vi "Keithley2450GateS.vi"() -> ()   [LabVIEW 2025]
doc: "Author: Scott Hannahs <sth@magnet.fsu.edu>\n\nThis software is licensed for use under the “MIT License\"\nCopyright (c) 2025 Scott Hannahs, sth@sth@magnet.sthnet.net\n\nPermission is hereby granted, free of charge, to any person obtaining a copy of this software and associated documentation files (the \"Software\"), to deal in the Software without restriction, including without limitation the rights to use, copy, modify, merge, publish, distribute, sublicense, and/or sell copies of the Software, and to permit persons to whom the Software is furnished to do so, subject to the following conditions: The above copyright notice and this permission notice shall be included in all copies or substantial portions of the Software.\n\nTHE SOFTWARE IS PROVIDED \"AS IS\", WITHOUT WARRANTY OF ANY KIND, EXPRESS OR IMPLIED, INCLUDING BUT NOT LIMITED TO THE WARRANTIES OF MERCHANTABILITY, FITNESS FOR A PARTICULAR PURPOSE AND NONINFRINGEMENT. IN NO EVENT SHALL THE AUTHORS OR COPYRIGHT HOLDERS BE LIABLE FOR ANY CLAIM, DAMAGES OR OTHER LIABILITY, WHETHER IN AN ACTION OF CONTRACT, TORT OR OTHERWISE, ARISING FROM, OUT OF OR IN CONNECTION WITH THE SOFTWARE OR THE USE OR OTHER DEALINGS IN THE SOFTWARE."
panel:
  out "Sweep\nTime  (sec)":u32 format="%.1f"
  in  "Button:SetupBySoft":bool
  in  "Autozero:":bool
  out "Was paused":bool=TRUE
  in  "VISA resource name":refnum<visa-resource-name>="GPIB0::15::INSTR"
  in  "INFINITE RUN":bool
  in  "MODE:":enum32{"SAW /|/|/|", "TRINGLE /\\/\\/\\"}(radio)=enum."TRINGLE /\\/\\/\\"
  in  "Step |Volt| (abs.)":dbl=0.05 min=1e-06 max=0.1 format="%^.3e"
  in  "Delay (s)":dbl=1.0 min=0.1 max=100.0 format="%.3f"
  in  "Stop Volt":dbl=1.0 min=-10.0 max=10.0 format="%^.3e"
  in  "Start Sweep":bool
  out "Last index":i32
  in  "Compliance Current":dbl=1e-07 format="%.3e"
  in  "Start Volt":dbl min=-10.0 max=10.0 format="%^.3e"
  in  "Setup":bool
  in  "Pause/Resume sweep":bool
  out "StartStorage":dbl min=-10.0 max=10.0 format="%^.3e"
  out "StopStorage":dbl=1.0 min=-10.0 max=10.0 format="%^.3e"
  in  "Button:Continue":bool
  in  "Button:SweepBySoft":bool
  out "Volt by Computer":dbl min=-10.0 max=10.0 format="%^.3e"
  in  "stop sweep":bool
  in  "Output Zero":bool
  # "Select name then start VI"
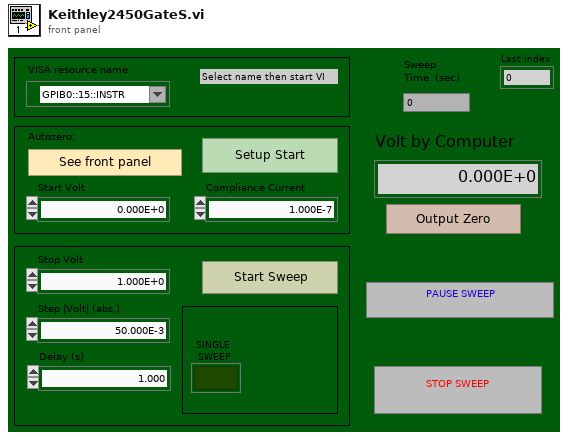
[diagram p1: front panel]
types:
  T1 = enum8{"Enabled", "Disabled", "Disabled and Grayed Out"}
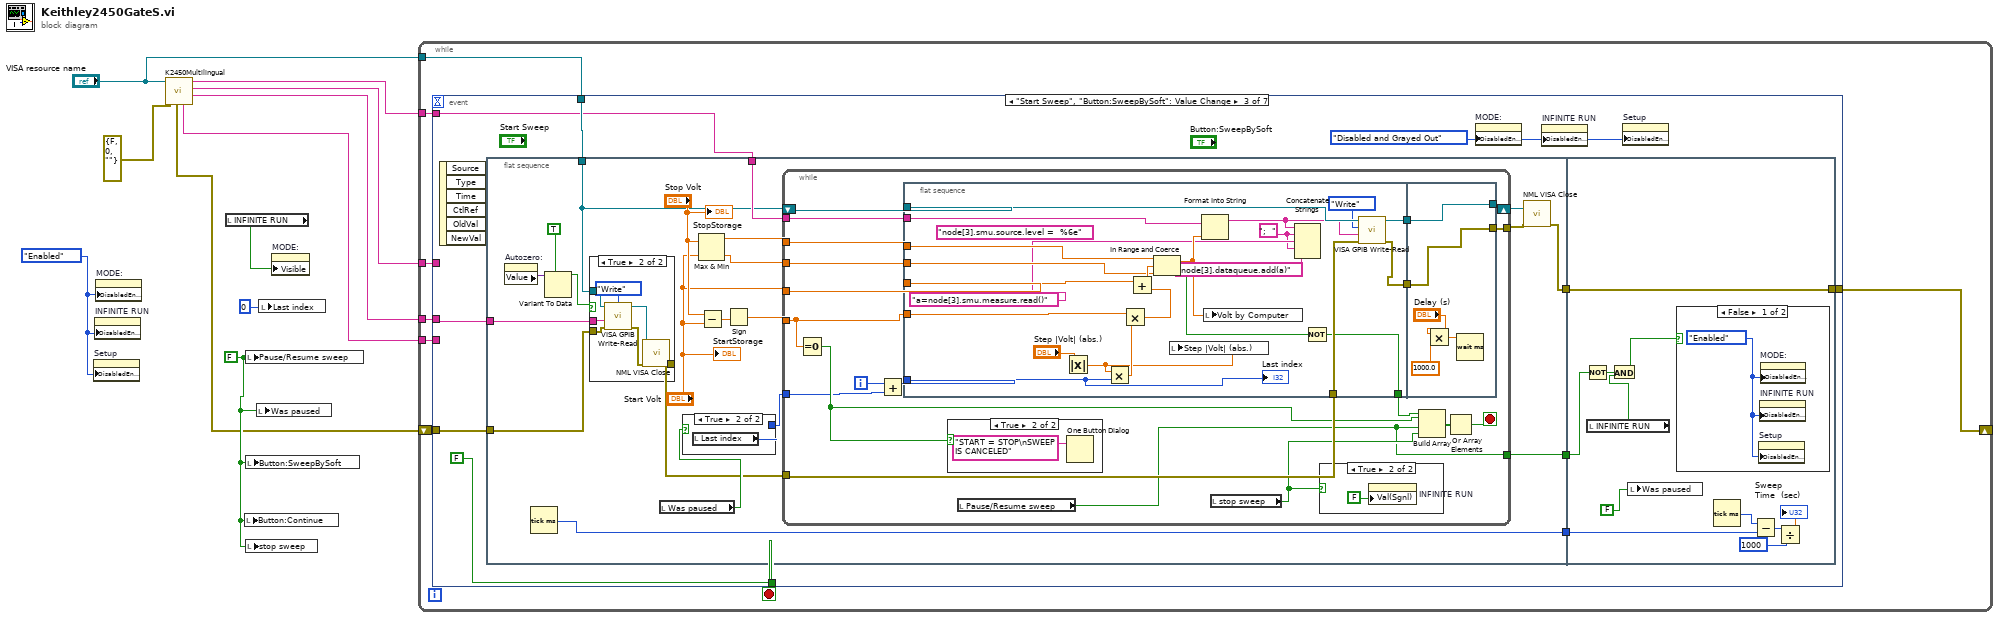
[diagram p0: block diagram]
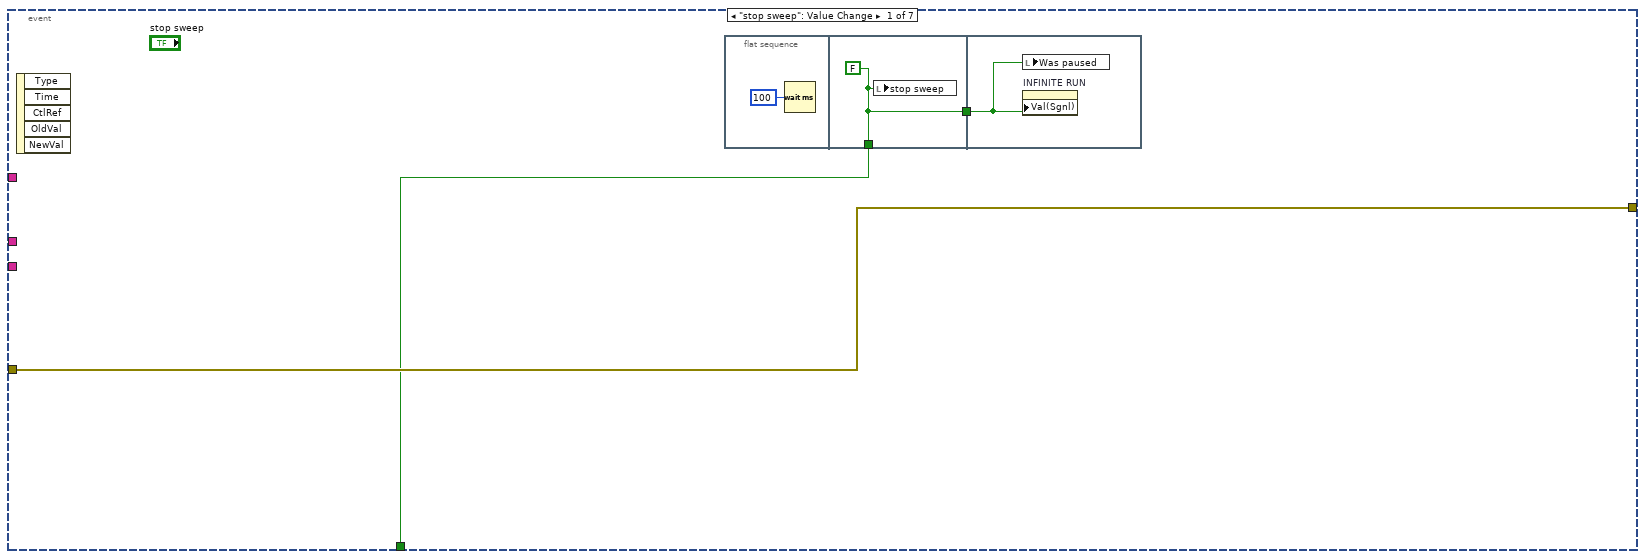
[diagram p2: hidden frame]
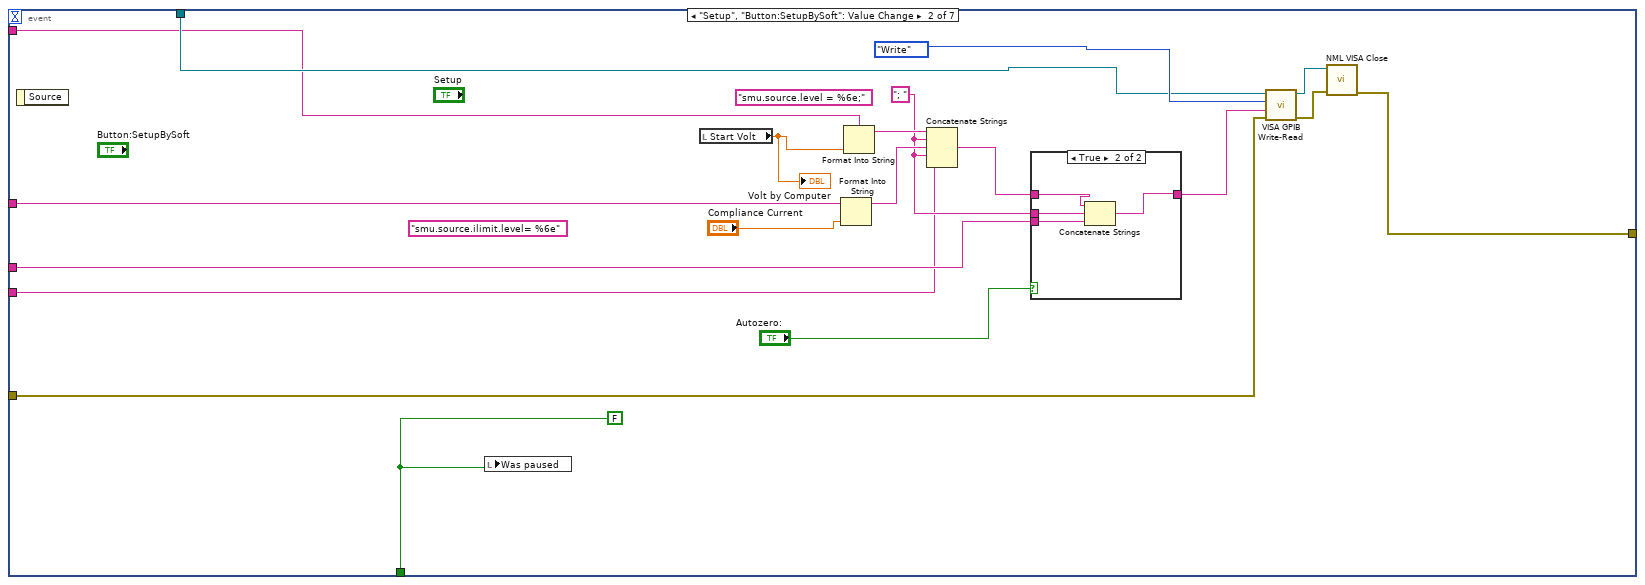
[diagram p3: hidden frame]
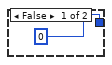
[diagram p6: hidden frame]
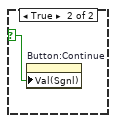
[diagram p9: hidden frame]
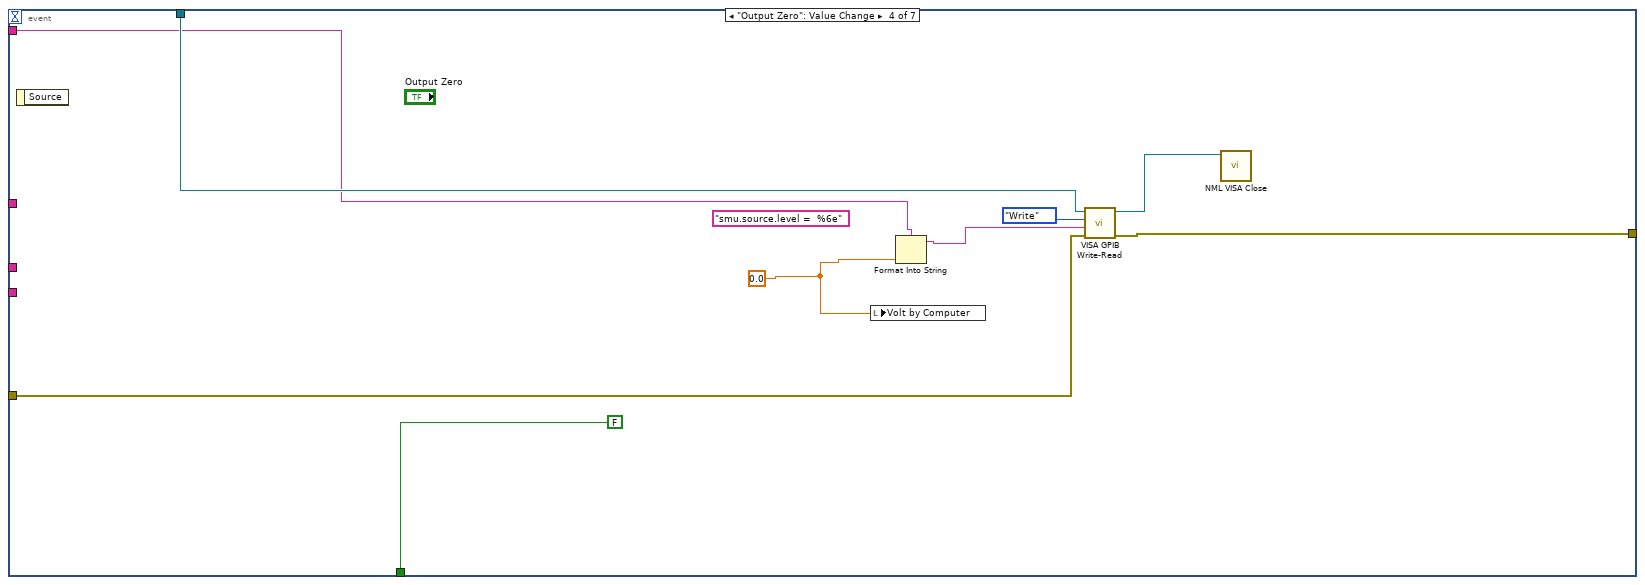
[diagram p10: hidden frame]
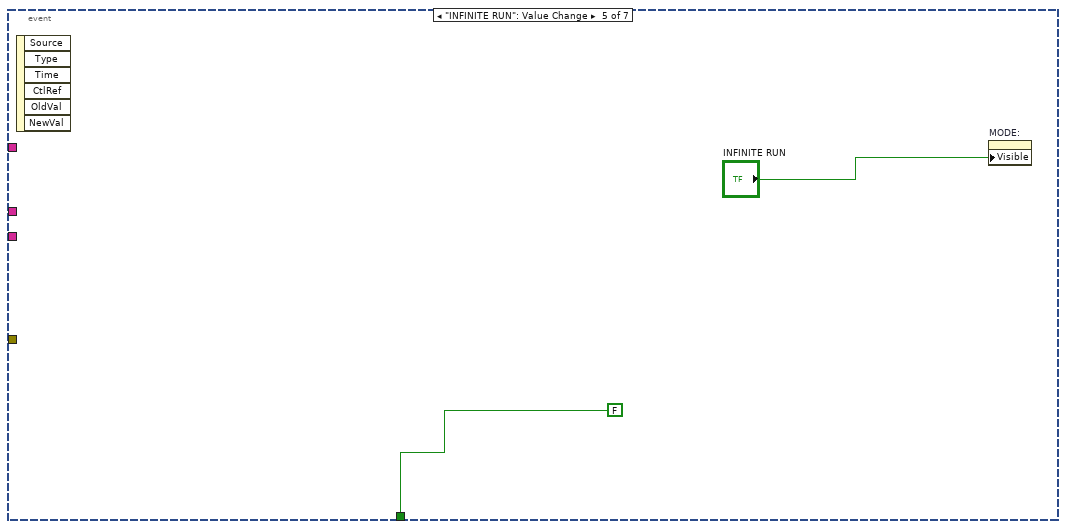
[diagram p11: hidden frame]
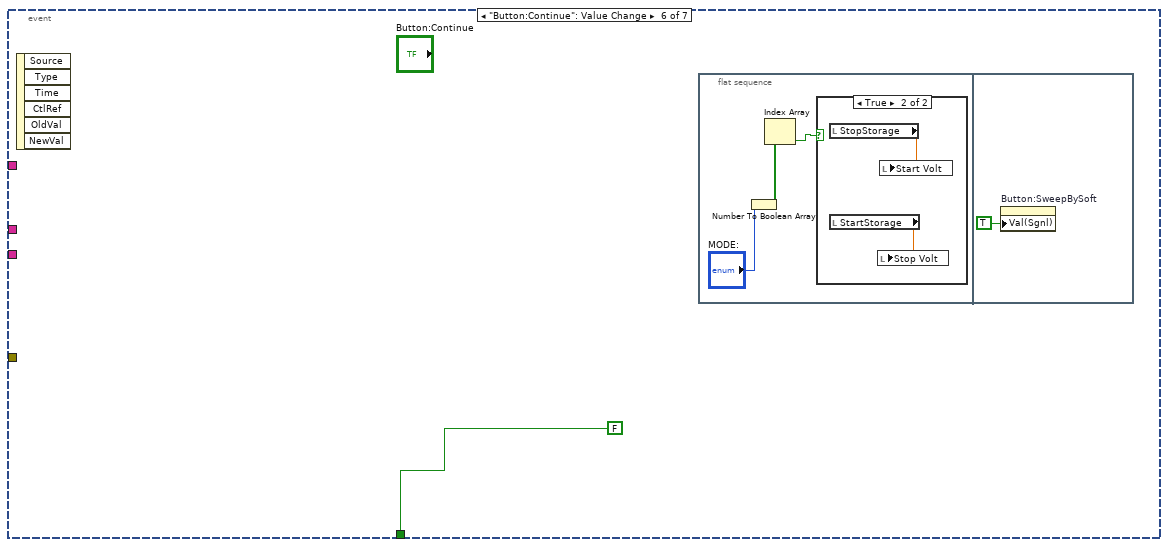
[diagram p12: hidden frame]
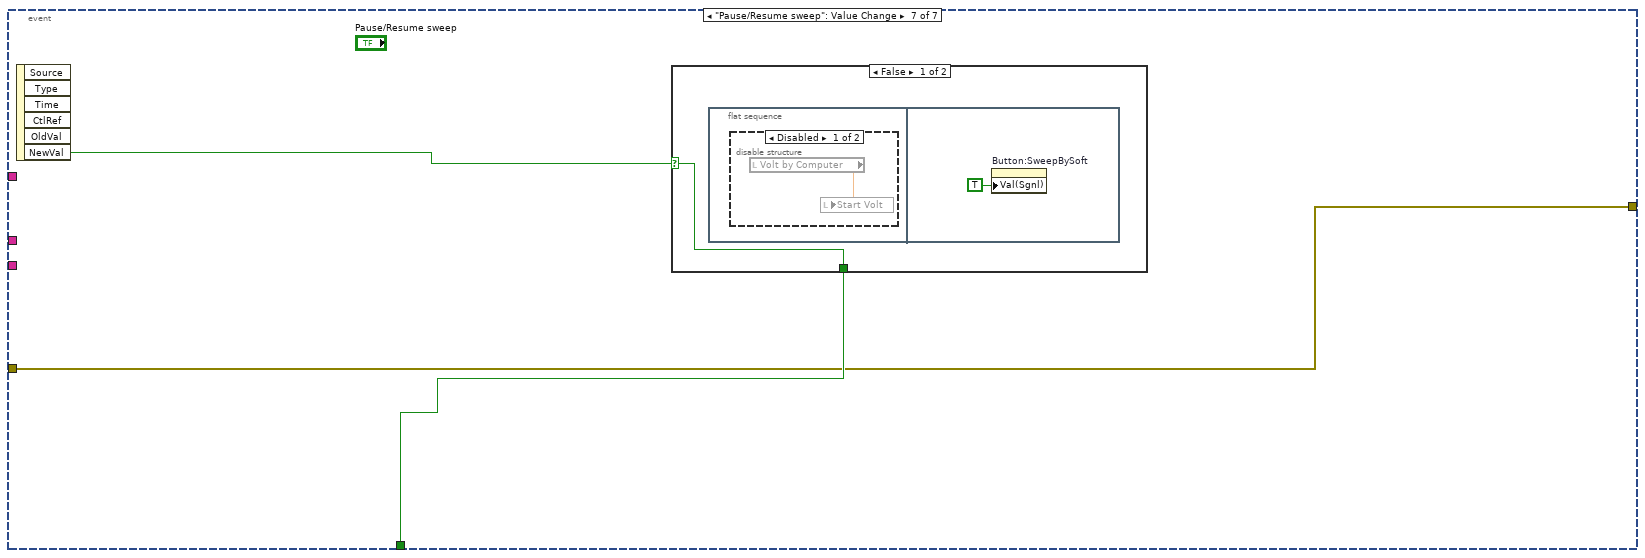
[diagram p14: hidden frame]
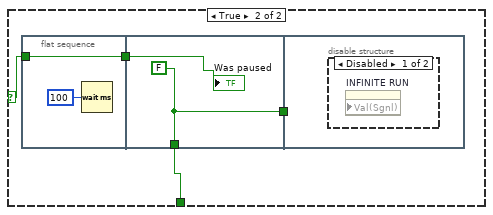
[diagram p16: hidden frame]
diagram:
  w8 = T1."Enabled" ("Disabled")
  w9 = FALSE ("Pause/Resume sweep")
  n1 = property on="Setup" class="Bool"("DisabledEnum"=w8) -> ()  [unwired: 2 in, 2 out]
  n2 = property on="INFINITE RUN" class="Bool (strict)"("DisabledEnum"=w8) -> ()  [unwired: 2 in, 2 out]
  n3 = property on="MODE:" class="RadioBtnsControl (strict)"("DisabledEnum"=w8) -> ()  [unwired: 2 in, 2 out]
  n4 = call "K2450Multilingual.vi"("error in"=errorcluster {"status"=FALSE, "code"=0, "source"=""} ("error out"), "VISA resource name"="VISA resource name") -> ("AutozeroOnce"=w3:string, "Set Compliance"=w4:string, "Set Source Level"=w5:string, "Clear defbuffer1"=w1:string, "error out"=w6:errorcluster)  [unwired: 2 in, 2 out]
  n5 = local read "INFINITE RUN"() -> (w11:bool)
  n6 = local write "Button:Continue"(w9) -> ()
  n7 = local write "Pause/Resume sweep"(w9) -> ()
  n8 = local write "Button:SweepBySoft"(w9) -> ()
  n9 = local write "stop sweep"(w9) -> ()
  n10 = local write "Was paused"(w9) -> ()
  n11 = local write "Last index"(0 ("Last index")) -> ()
  n12 = property on="MODE:" class="RadioBtnsControl (strict)"("Visible"=w11) -> ()  [unwired: 2 in, 2 out]
  n13 = while {
    shift-right: [w18] -> _
    shift-left: w6 -> [w17]
    tunnel: "VISA resource name" -> [w16]
    tunnel: w5 -> [w15]
    tunnel: w4 -> [w14]
    tunnel: w3 -> [w13]
    tunnel: w1 -> [w12]
    stop <- w19 stop-if-true
    n14 = event shown="[2] \"Start Sweep\", \"Button:SweepBySoft\": Value Change" {
      selector: _ -> [_ _ _ _ _ _ _]
      dyn-events: _ -> [_ _ _ _ _ _ _]
      timeout: _ -> [_ _ _ _ _ _ _]
      tunnel: w16 -> [_ w38 w59 w161 _ _ _]
      tunnel: [w21 w36 FALSE ("NewVal") FALSE ("NewVal") FALSE ("NewVal") FALSE ("NewVal") w174] -> w19
      tunnel: [w22 w40 w57 w160 _ _ w173] -> w18
      tunnel: w17 -> [w22 w37 w58 w159 _ _ w173]
      tunnel: w15 -> [_ w34 w52 w154 _ _ _]
      tunnel: w14 -> [_ w33 _ _ _ _ _]
      tunnel: w13 -> [_ w30 w51 _ _ _ _]
      tunnel: w12 -> [_ w26 _ _ _ _ _]
      event "stop sweep": Value Change {
        n15 = event-data() -> ()  [unwired: 1 in, 5 out]
        n16 = flat-sequence {
          tunnel: [w24] -> w21
          tunnel: [w24] -> w20
          tunnel: w20 -> [w25]
          frame #0 {
            n17 = Wait (ms)(milliseconds to wait=u32 100) -> ()  [unwired: 1 out]
          }
          frame #1 {
            w24 = FALSE ("stop")
            n18 = local write "stop sweep"(w24) -> ()
          }
          frame #2 {
            n19 = local write "Was paused"(w25) -> ()
            n20 = property on="INFINITE RUN" class="Bool (strict)"("Val(Sgnl)"=w25) -> ()  [unwired: 2 in, 2 out]
          }
        }
      }
      event "Setup", "Button:SetupBySoft": Value Change {
        (unwired) "smu.source.ilimit.level= %6e"
        w27 = "; " ("string")
        w36 = FALSE ("NewVal")
        (unwired) "smu.source.level = %6e;"
        n21 = event-data() -> ()  [unwired: 1 in, 1 out]
        n22 = local write "Was paused"(w36) -> ()
        n23 = local read "Start Volt"() -> (w44:dbl)
        "Volt by Computer" <- w44
        n24 = Format Into String(format string=w33, "Compliance Current") -> (resulting string=w35:string)  [unwired: 2 in, 1 out]
        n25 = Format Into String(format string=w34, w44) -> (resulting string=w29:string)  [unwired: 2 in, 1 out]
        n26 = Concatenate Strings(w29, w27, w35, w27, w26) -> (w28:string)
        n27 = case shown="True" "Autozero:" {
          tunnel: w28 -> [w45 w49]
          tunnel: [w45 w46] -> w31
          tunnel: w27 -> [_ w48]
          tunnel: w30 -> [_ w47]
          frame False {
          }
          frame True {
            n28 = Concatenate Strings(w49, w48, w47) -> (w46:string)
          }
        }
        n29 = call "VISA GPIB Write-Read.vi"("error in (no error)"=w37, "Command"=w31, "Action"=enum16{"Write", "Read", "Write & Read"}."Write", "VISA resource name"=w38) -> ("error out"=w41:errorcluster, "dup VISA Session"=w42:refnum<visa-resource-name>)  [unwired: 4 in, 2 out]
        n30 = call "NML VISA Close.vi"("Error In"=w41, "VISA resource name"=w42) -> ("Error Out"=w40:errorcluster)  [unwired: 9 in]
      }
      event "Start Sweep", "Button:SweepBySoft": Value Change {
        w53 = T1."Disabled and Grayed Out" ("Disabled")
        n31 = event-data() -> ()  [unwired: 1 in, 6 out]
        n32 = flat-sequence {
          tunnel: w59 -> [w64]
          tunnel: [w74] -> w55
          tunnel: [w69] -> w54
          tunnel: w52 -> [w68]
          tunnel: w58 -> [w67]
          tunnel: w51 -> [w65]
          tunnel: [w60] -> w50
          tunnel: [w151] -> w57
          tunnel: w55 -> [w151]
          tunnel: w54 -> [w147]
          tunnel: w50 -> [w141]
          frame #0 {
            n33 = property on="Autozero:" class="Bool"() -> ("Value"=w63:variant)  [unwired: 2 in, 2 out]
            n34 = Tick Count (ms)() -> (millisecond timer value=w60:u32)
            n35 = Variant To Data(type=TRUE, Variant=w63) -> (data=w61:bool)  [unwired: 1 in, 1 out]
            n36 = case shown="True" w61 {
              tunnel: w67 -> [w81 w87]
              tunnel: [w81 w85] -> w66
              tunnel: w65 -> [_ w84]
              tunnel: w64 -> [_ w82]
              frame False {
              }
              frame True {
                n37 = call "VISA GPIB Write-Read.vi"("error in (no error)"=w87, "Command"=w84, "Action"=enum16{"Write", "Read", "Write & Read"}."Write", "VISA resource name"=w82) -> ("error out"=w86:errorcluster, "dup VISA Session"=w83:refnum<visa-resource-name>)  [unwired: 4 in, 2 out]
                n38 = call "NML VISA Close.vi"("Error In"=w86, "VISA resource name"=w83) -> ("Error Out"=w85:errorcluster)  [unwired: 9 in]
              }
            }
            n39 = local read "Was paused"() -> (w71:bool)
            n40 = case shown="True" w71 {
              tunnel: [0 w90] -> w70
              frame False {
              }
              frame True {
                n41 = local read "Last index"() -> (w90:i32)
              }
            }
            n42 = Max & Min(x="Stop Volt", y="Start Volt") -> (max(x,y)=w80:dbl, min(x,y)=w79:dbl)
            n43 = Subtract(x="Stop Volt", y="Start Volt") -> (x-y=w76:dbl)
            n44 = Sign(1:w76) -> (0:w75:dbl)
            n45 = while {
              tunnel: w66 -> [w110]
              tunnel: "Start Volt" -> [w109]
              tunnel: w80 -> [w104]
              tunnel: w79 -> [w103]
              tunnel: w75 -> [w97]
              tunnel: [w101] -> w73
              shift-right: [w100] -> w72
              shift-left: w64 -> [w99]
              tunnel: w70 -> [w94]
              tunnel: [w92] -> w69
              tunnel: w68 -> [w91]
              i -> [w107]
              stop <- w106 stop-if-true
              n46 = Equal To 0?(x=w97) -> (x = 0?=w96:bool)
              n47 = Add(x=w107, y=w94) -> (x+y=w98:i32)
              n48 = flat-sequence {
                tunnel: w99 -> [w135]
                tunnel: w110 -> [w134]
                tunnel: w109 -> [w132]
                tunnel: [w129] -> w105
                tunnel: [w133] -> w108
                tunnel: w98 -> [w118]
                tunnel: w104 -> [w124]
                tunnel: w103 -> [w123]
                tunnel: w97 -> [w120]
                tunnel: [w119] -> w102
                tunnel: w91 -> [w114]
                tunnel: w108 -> [w137]
                tunnel: w102 -> [w136]
                tunnel: [w137] -> w101
                tunnel: [w136] -> w100
                frame #0 {
                  w116 = ";  " ("string")
                  (unwired) "node[3].smu.source.level =  %6e"
                  n49 = Absolute Value(x="Step |Volt| (abs.)") -> (abs(x)=w122:dbl)
                  n50 = Multiply(x=w122, y=w118) -> (x*y=w126:dbl)
                  n51 = Multiply(x=w120, y=w126) -> (x*y=w121:dbl)
                  n52 = Add(x=w132, y=w121) -> (x+y=w131:dbl)
                  n53 = In Range and Coerce(upper limit=w124, x=w131, lower limit=w123) -> (coerced(x)=w125:dbl, In Range?=w130:bool)
                  n54 = local write "Step |Volt| (abs.)"(w122) -> ()
                  n55 = Format Into String(format string=w114, w125) -> (resulting string=w113:string)  [unwired: 2 in, 1 out]
                  n56 = local write "Volt by Computer"(w125) -> ()
                  n57 = Concatenate Strings(w113, w116, "a=node[3].smu.measure.read()" ("string"), w116, "node[3].dataqueue.add(a)" ("string")) -> ()  [unwired: 1 out]
                  n58 = Not(x=w130) -> (.not. x?=w129:bool)
                  n59 = call "VISA GPIB Write-Read.vi"("error in (no error)"=w134, "Command"=w113, "Action"=enum16{"Write", "Read", "Write & Read"}."Write", "VISA resource name"=w135) -> ("error out"=w133:errorcluster, "dup VISA Session"=w119:refnum<visa-resource-name>)  [unwired: 4 in, 2 out]
                  "Last index" <- w118
                }
                frame #1 {
                  n60 = Multiply(x="Delay (s)", y=1000.0) -> (x*y=w139:dbl)
                  n61 = Wait (ms)(milliseconds to wait=w139) -> ()  [unwired: 1 out]
                }
              }
              n62 = case shown="True" w96 {
                frame False {
                }
                frame True {
                  n63 = One Button Dialog(message="START = STOP\nSWEEP IS CANCELED") -> ()  [unwired: 1 in, 1 out]
                }
              }
              n64 = local read "Pause/Resume sweep"() -> (w92:bool)
              n65 = local read "stop sweep"() -> (w93:bool)
              n66 = case shown="True" w93 {
                frame False {
                }
                frame True {
                  n67 = property on="INFINITE RUN" class="Bool (strict)"("Val(Sgnl)"=FALSE ("Value (Signaling)")) -> ()  [unwired: 2 in, 2 out]
                }
              }
              n68 = Build Array(w105, w96, w92, w93) -> (w95:bool[])
              n69 = Or Array Elements(Boolean array=w95) -> (logical OR=w106:bool)
            }
            n70 = call "NML VISA Close.vi"("Error In"=w73, "VISA resource name"=w72) -> ("Error Out"=w74:errorcluster)  [unwired: 9 in]
            "StopStorage" <- "Stop Volt"
            "StartStorage" <- "Start Volt"
          }
          frame #1 {
            n71 = Not(x=w147) -> (.not. x?=w146:bool)
            n72 = local read "INFINITE RUN"() -> (w150:bool)
            n73 = And(x=w146, y=w150) -> (x .and. y?=w148:bool)
            n74 = local write "Was paused"(FALSE) -> ()
            n75 = case shown="False" w148 {
              selector: w148 -> [_ w153]
              frame False {
                w152 = T1."Enabled" ("Disabled")
                n76 = property on="Setup" class="Bool"("DisabledEnum"=w152) -> ()  [unwired: 2 in, 2 out]
                n77 = property on="INFINITE RUN" class="Bool (strict)"("DisabledEnum"=w152) -> ()  [unwired: 2 in, 2 out]
                n78 = property on="MODE:" class="RadioBtnsControl (strict)"("DisabledEnum"=w152) -> ()  [unwired: 2 in, 2 out]
              }
              frame True {
                n79 = property on="Button:Continue" class="Bool (strict)"("Val(Sgnl)"=w153) -> ()  [unwired: 2 in, 2 out]
              }
            }
            n80 = Tick Count (ms)() -> (millisecond timer value=w145:u32)
            n81 = Subtract(x=w145, y=w141) -> (x-y=w143:u32)
            n82 = Divide(x=w143, y=u32 1000) -> (x/y=→"Sweep\nTime  (sec)":dbl)
          }
        }
        n83 = property on="MODE:" class="RadioBtnsControl (strict)"("DisabledEnum"=w53) -> ()  [unwired: 2 in, 2 out]
        n84 = property on="INFINITE RUN" class="Bool (strict)"("DisabledEnum"=w53) -> ()  [unwired: 2 in, 2 out]
        n85 = property on="Setup" class="Bool"("DisabledEnum"=w53) -> ()  [unwired: 2 in, 2 out]
      }
      event "Output Zero": Value Change {
        w156 = 0.0 ("Output Volt 2")
        (unwired) "smu.source.level =  %6e"
        n86 = event-data() -> ()  [unwired: 1 in, 1 out]
        n87 = local write "Volt by Computer"(w156) -> ()
        n88 = Format Into String(format string=w154, w156) -> (resulting string=w157:string)  [unwired: 2 in, 1 out]
        n89 = call "VISA GPIB Write-Read.vi"("error in (no error)"=w159, "Command"=w157, "Action"=enum16{"Write", "Read", "Write & Read"}."Write", "VISA resource name"=w161) -> ("error out"=w160:errorcluster, "dup VISA Session"=w155:refnum<visa-resource-name>)  [unwired: 4 in, 2 out]
        n90 = call "NML VISA Close.vi"("VISA resource name"=w155) -> ()  [unwired: 10 in, 1 out]
      }
      event "INFINITE RUN": Value Change {
        n91 = event-data() -> ()  [unwired: 1 in, 6 out]
        n92 = property on="MODE:" class="RadioBtnsControl (strict)"("Visible"="INFINITE RUN") -> ()  [unwired: 2 in, 2 out]
      }
      event "Button:Continue": Value Change {
        n93 = event-data() -> ()  [unwired: 1 in, 6 out]
        n94 = flat-sequence {
          frame #0 {
            n95 = Number To Boolean Array(number="MODE:") -> (Boolean array=w168:bool[])
            n96 = Index Array(array=w168) -> (element=w166:bool)  [unwired: 1 in]
            n97 = case shown="True" w166 {
              frame False {
              }
              frame True {
                n98 = local read "StopStorage"() -> (w170:dbl)
                n99 = local read "StartStorage"() -> (w169:dbl)
                n100 = local write "Stop Volt"(w169) -> ()
                n101 = local write "Start Volt"(w170) -> ()
              }
            }
          }
          frame #1 {
            n102 = property on="Button:SweepBySoft" class="Bool (strict)"("Val(Sgnl)"=TRUE ("Value (Signaling)")) -> ()  [unwired: 2 in, 2 out]
          }
        }
      }
      event "Pause/Resume sweep": Value Change {
        n103 = event-data() -> ("NewVal"=w172:bool)  [unwired: 1 in, 5 out]
        n104 = case shown="False" w172 {
          selector: w172 -> [w175 w178]
          tunnel: [w175 w180] -> w174
          frame False {
            n105 = flat-sequence {
              frame #0 {
                n106 = disable-structure shown="Disabled" {
                  frame Disabled {
                    n107 = local read "Volt by Computer"() -> (w176:dbl)
                    n108 = local write "Start Volt"(w176) -> ()
                  }
                  frame Enabled {
                  }
                }
              }
              frame #1 {
                n109 = property on="Button:SweepBySoft" class="Bool (strict)"("Val(Sgnl)"=TRUE ("Value (Signaling)")) -> ()  [unwired: 2 in, 2 out]
              }
            }
          }
          frame True {
            n110 = flat-sequence {
              tunnel: [w182] -> w179
              tunnel: w178 -> [w182]
              tunnel: [w185] -> w180
              tunnel: [w185] -> w181
              tunnel: w179 -> [w184]
              tunnel: w181 -> [_]
              frame #0 {
                n111 = Wait (ms)(milliseconds to wait=u32 100) -> ()  [unwired: 1 out]
              }
              frame #1 {
                w185 = FALSE ("stop")
                "Was paused" <- w184
              }
              frame #2 {
                n112 = disable-structure shown="Disabled" {
                  frame Disabled {
                    n113 = property on="INFINITE RUN" class="Bool (strict)" props=["Val(Sgnl)"]() -> ()  [unwired: 3 in, 2 out]
                  }
                  frame Enabled {
                  }
                }
              }
            }
          }
        }
      }
    }
  }
